vi "vent_valve_control.vi"(10 "Flow Rate":dbl, 11 "physical channels":tag) -> ()   [LabVIEW 2014]
uses:
  <vilib>/DAQmx/create/channels.llb/DAQmx Create Channel (AO-Voltage-Basic).vi
  <vilib>/DAQmx/write.llb/DAQmx Write (Analog DBL 1Chan 1Samp).vi
panel:
  in  "timeout":dbl=10.0 format="%0.2f"
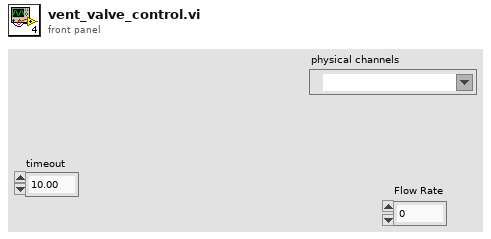
[diagram p1: front panel]
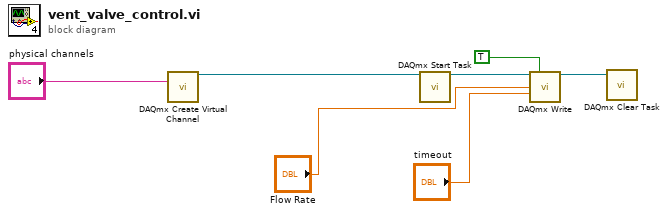
[diagram p0: block diagram]
diagram:
  n1 = call-poly <vilib>:"DAQmx Create Virtual Channel.vi"("physical channels"="physical channels") -> ("task out"=w2:refnum<k21>)  [unwired: 13 in, 1 out]
  n2 = call <vilib>:"DAQmx Start Task.vi"("task/channels in"=w2) -> ("task out"=w6:refnum<k21>)  [unwired: 13 in, 1 out]
  n3 = call-poly <vilib>:"DAQmx Write.vi"("task/channels in"=w6, "auto start"=TRUE, "data"="Flow Rate", "timeout"="timeout") -> ("task out"=w3:refnum<k21>)  [unwired: 9 in, 2 out]
  n4 = call <vilib>:"DAQmx Clear Task.vi"("task in"=w3) -> ()  [unwired: 14 in, 1 out]
